vi "Hide window.vi"(0 "LV MDI in":refnum<class "LV MDI.lvclass">, 5 "Doc Name[]":string[](array[string]), 11 "error in (no error)":errorcluster) -> (4 "LV MDI out":refnum<class "LV MDI.lvclass">, 15 "error out":errorcluster)   [LabVIEW 2016, in "LV MDI.lvclass"]
doc: "Hides the window."
uses:
  LV MDI.lvclass
  LV MDI.lvclass/LV MDI.ctl
  Document/Document.lvclass/Document.ctl
  user32.dll
  Document/Document.lvclass
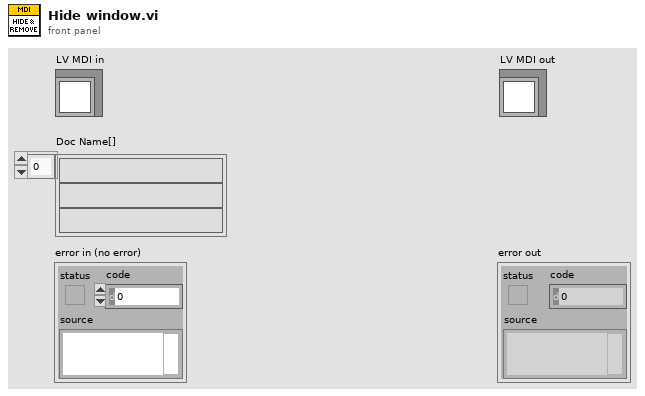
[diagram p1: front panel]
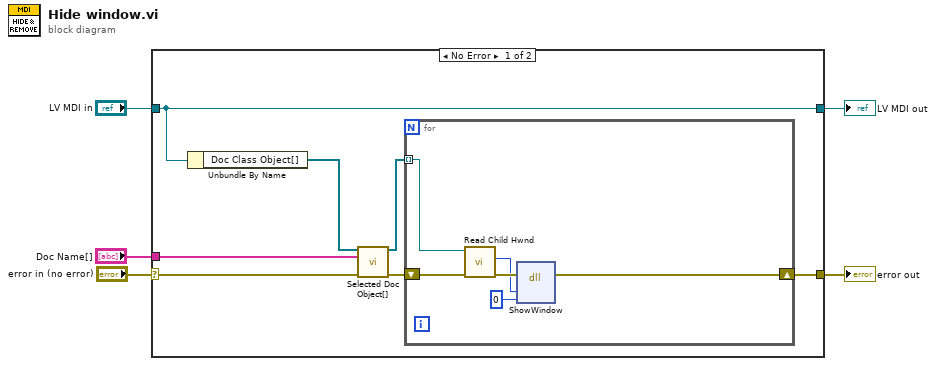
[diagram p0: block diagram]
diagram:
  n1 = case shown="No Error" "error in (no error)" {
    selector: "error in (no error)" -> [w10 w20]
    tunnel: [w12 w20] -> w4
    tunnel: [w11 w19] -> w2
    tunnel: "LV MDI in" -> [w11 w19]
    tunnel: "Doc Name[]" -> [w6 _]
    frame No Error {
      n2 = Unbundle By Name(w11) -> ("Doc Class Object[]"=w8:refnum<class "Document.lvclass">[])
      n3 = call "Selected Doc Object[].vi"("Doc Class Object[]"=w8, "Doc Name[]"=w6, "error in"=w10) -> ("Selected Doc[]"=w7:refnum<class "Document.lvclass">[], "error Out"=w9:errorcluster)  [unwired: 11 in]
      n4 = for {
        shift-right: [w18] -> w12
        shift-left: w9 -> [w16]
        tunnel: w7 -> [w13] mode=indexing
        n5 = call "Read Child Hwnd.vi"("error in (no error)"=w16, "Document in"=w13) -> ("error out"=w15:errorcluster, "Child Hwnd"=w14:u32)  [unwired: 7 in, 1 out]
        n6 = dll-call lib="user32.dll" fn="ShowWindow"(error in=w15, "hwnd"=w14, "nCmdShow"=u32 0) -> (error out=w18:errorcluster)  [unwired: 5 in, 1 out]
      }
    }
    frame Error {
    }
  }
  "error out" <- w4
  "LV MDI out" <- w2
